vi "Trigger Scope.vi"(8 "error in (no error)":errorcluster) -> (0 "error out":errorcluster)   [LabVIEW 2019]
uses:
  <vilib>/Rock Robotics/SystemInterfaces/DIO/FPGA_DIOChannel.ctl
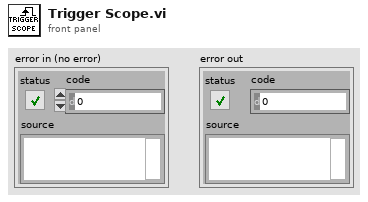
[diagram p1: front panel]
types:
  T1 = typedef "WPI_DigitalOutputDevRef.ctl" = cluster{"DIO Channel":T2, "DevStatus":errorcluster}
  T2 = typedef "FPGA_DIOChannel.ctl" = enum8{"DIO 0", "DIO 1", "DIO 2", "DIO 3", "DIO 4", "DIO 5", "DIO 6", "DIO 7", "DIO 8", "DIO 9", "DIO MXP 0", "DIO MXP 1", "DIO MXP 2", "DIO MXP 3", "DIO MXP 4", "DIO MXP 5", "DIO MXP 6", "DIO MXP 7", "DIO MXP 8", "DIO MXP 9", "DIO MXP 10", "DIO MXP 11", "DIO MXP 12", "DIO MXP 13", "DIO MXP 14", "DIO MXP 15", "SPI Port CS1", "SPI Port CS2", "SPI Port CS3", "SPI Port MISO", "SPI Port MOSI", "Invalid"}
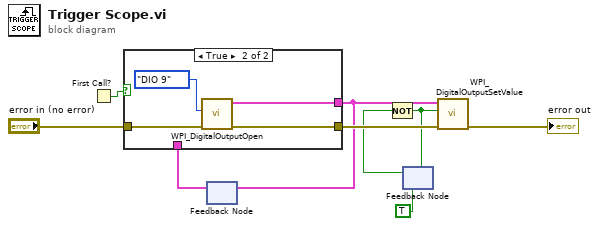
[diagram p0: block diagram]
diagram:
  n1 = First Call?() -> (First Call?: T/F=w4:bool)
  n2 = feedback #1() -> (w5:T1)  [unwired: 1 in]
  n3 = case shown="True" w4 {
    tunnel: "error in (no error)" -> [w10 w15]
    tunnel: [w11 w14] -> w6
    tunnel: [w10 w13] -> w7
    tunnel: w5 -> [w11 _]
    frame False {
    }
    frame True {
      n4 = call <vilib>:"WPI_DigitalOutputOpen.vi"("error in (no error)"=w15, "DIO Channel"=FPGA_DIOChannel."DIO 9") -> ("error out"=w13:errorcluster, "DigitalOutputDevRef"=w14:T1)  [unwired: 8 in]
    }
  }
  n5 = feedback-in #1(w6) -> ()
  n6 = feedback #2(TRUE ("Value")) -> (w2:bool)
  n7 = Not(x=w2) -> (.not. x?=w1:bool)
  n8 = feedback-in #2(w1) -> ()
  n9 = call <vilib>:"WPI_DigitalOutputSetValue.vi"("error in (no error)"=w7, "Value"=w1, "DigitalOutputDevRef"=w6) -> ("error out"=→"error out":errorcluster)  [unwired: 7 in, 1 out]
